vi "Get_Parameter Json.vi"(8 "error in (no error)":errorcluster caption="entrée d'erreur (pas d'erreur)", 11 "Class Instrument (Default) en entrée":refnum<class "Class Instrument Printer.lvclass">) -> (0 "error out":errorcluster caption="sortie d'erreur", 2 "Parameter Json":string, 3 "Class Instrument (Default) en sortie":refnum<class "Class Instrument Printer.lvclass">)   [LabVIEW 2020, in "Library Instrument & Equipement.lvlib" / "Library Instruments.lvlib" / "Class Instrument Printer.lvclass"]
uses:
  Class Instrument Printer.lvclass
  Commun VI/TypeDef/Commande Printer/Commande Parameter Printer.ctl
  Printer/Printer (Default)/Class Printer (Default).lvclass
  Class Instrument Printer.lvclass/Class Instrument Printer.ctl
  JSON API/Variant JSON/Variant to JSON.vi
  JSON API/JSON Value/Get Item by name array.vi
  Instrument (Default)/Class Instrument (Default).lvclass
  JSON API/JSON Value/JSON Value.lvclass
  JSON API/Get Polymorphic/JSON GetSet.lvlib
  JSON API/Variant JSON/Variant JSON.lvlib
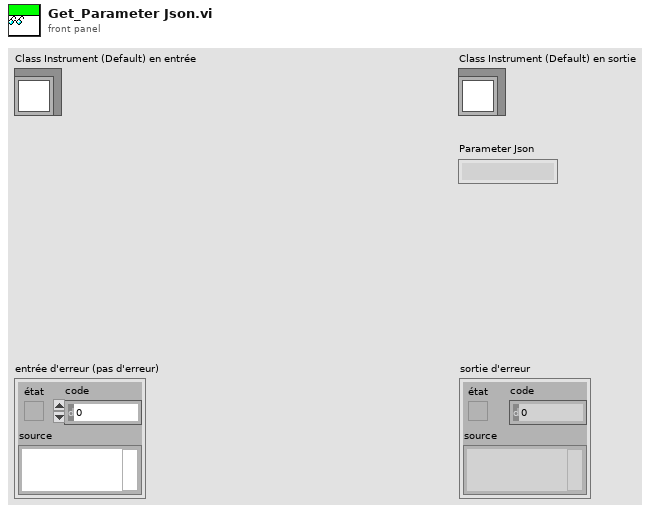
[diagram p1: front panel]
types:
  T1 = typedef "Commande Parameter Printer.ctl" = cluster{"Device_Printer":string, "File To print":path, "Path Picture":path, "Library Printer":refnum<class "Class Printer (Default).lvclass">}
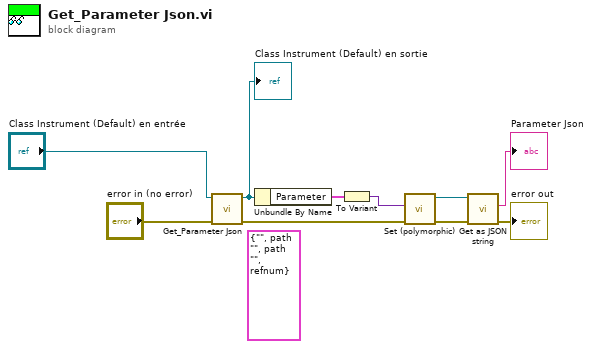
[diagram p0: block diagram]
diagram:
  (unwired) T1 {"Device_Printer"="", "File To print"=path "", "Path Picture"=path "", "Library Printer"=refnum} ("Parameter")
  n1 = call-parent "Get_Parameter Json.vi"("error in (no error)"="error in (no error)", "Class Instrument (Default) en entrée"="Class Instrument (Default) en entrée") -> ("error out"=w4:errorcluster, "Class Instrument (Default) en sortie"=w1:refnum<class "Class Instrument Printer.lvclass">)  [unwired: 7 in, 1 out]
  "Class Instrument (Default) en sortie" <- w1
  n2 = Unbundle By Name(w1) -> ("Parameter"=w5:T1)
  n3 = To Variant(anything=w5) -> (Variant=w8:variant)
  n4 = call-poly "Set (polymorphic).vi"("error in (no error)"=w4, "Variant"=w8) -> ("error out"=w6:errorcluster, "JSON Value out"=w7:refnum<class "JSON Value.lvclass">)  [unwired: 8 in]
  n5 = call "Get as JSON string.vi"("error in (no error)"=w6, "JSON Value in"=w7) -> ("error out"=→"error out":errorcluster, "<JSON>"=→"Parameter Json":string)  [unwired: 8 in]
